vi "HapticSPM_force_only.vi"() -> ()   [LabVIEW 2023]
uses:
  HapticSPM_write Folder/Program Files/National Instruments/LabVIEW 2022/user.lib/Haptic Prog Interface/Haptic Prog Interface.lvlib
  Haptic-Programming-Interface/src/x64/Debug/Haptic Programming Interface.dll
panel:
  out "Potential vs Distance":cluster{dbl[], dbl[]}(graph)
  out "Force vs Distance":cluster{dbl[], dbl[]}(graph)
  in  "Suggested Settings":bool=TRUE
  out "Z-Position":dbl caption="Numeric" format="%#.17p"
  out "Force":dbl(knob) scale=-3.0..3.0
  in  "Function":string(combo)="2" caption="Combo Box"
  in  "k":dbl=1.0 caption="Numeric" step=0.1 format="%.1g"
  in  "Setpoint":dbl=1e-10 caption="Numeric" step=1e-11 format="%.0p"
  in  "Gain":dbl=1.0 caption="Numeric" format="%.1g"
  # "Super Ultra Mega Haptic SPM Controller 3000"
  # "Signal"
  # "Height"
  # "Force"
  # "Force"
  # "Move pen in all three dimensions to calibrate before feeling surface\n\nClick \"enter\" to turn off recommended settings\n\nChange \"Setpoint\" and \"k\" parameters to adjust the feel of the force"
  # "Surface Scale"
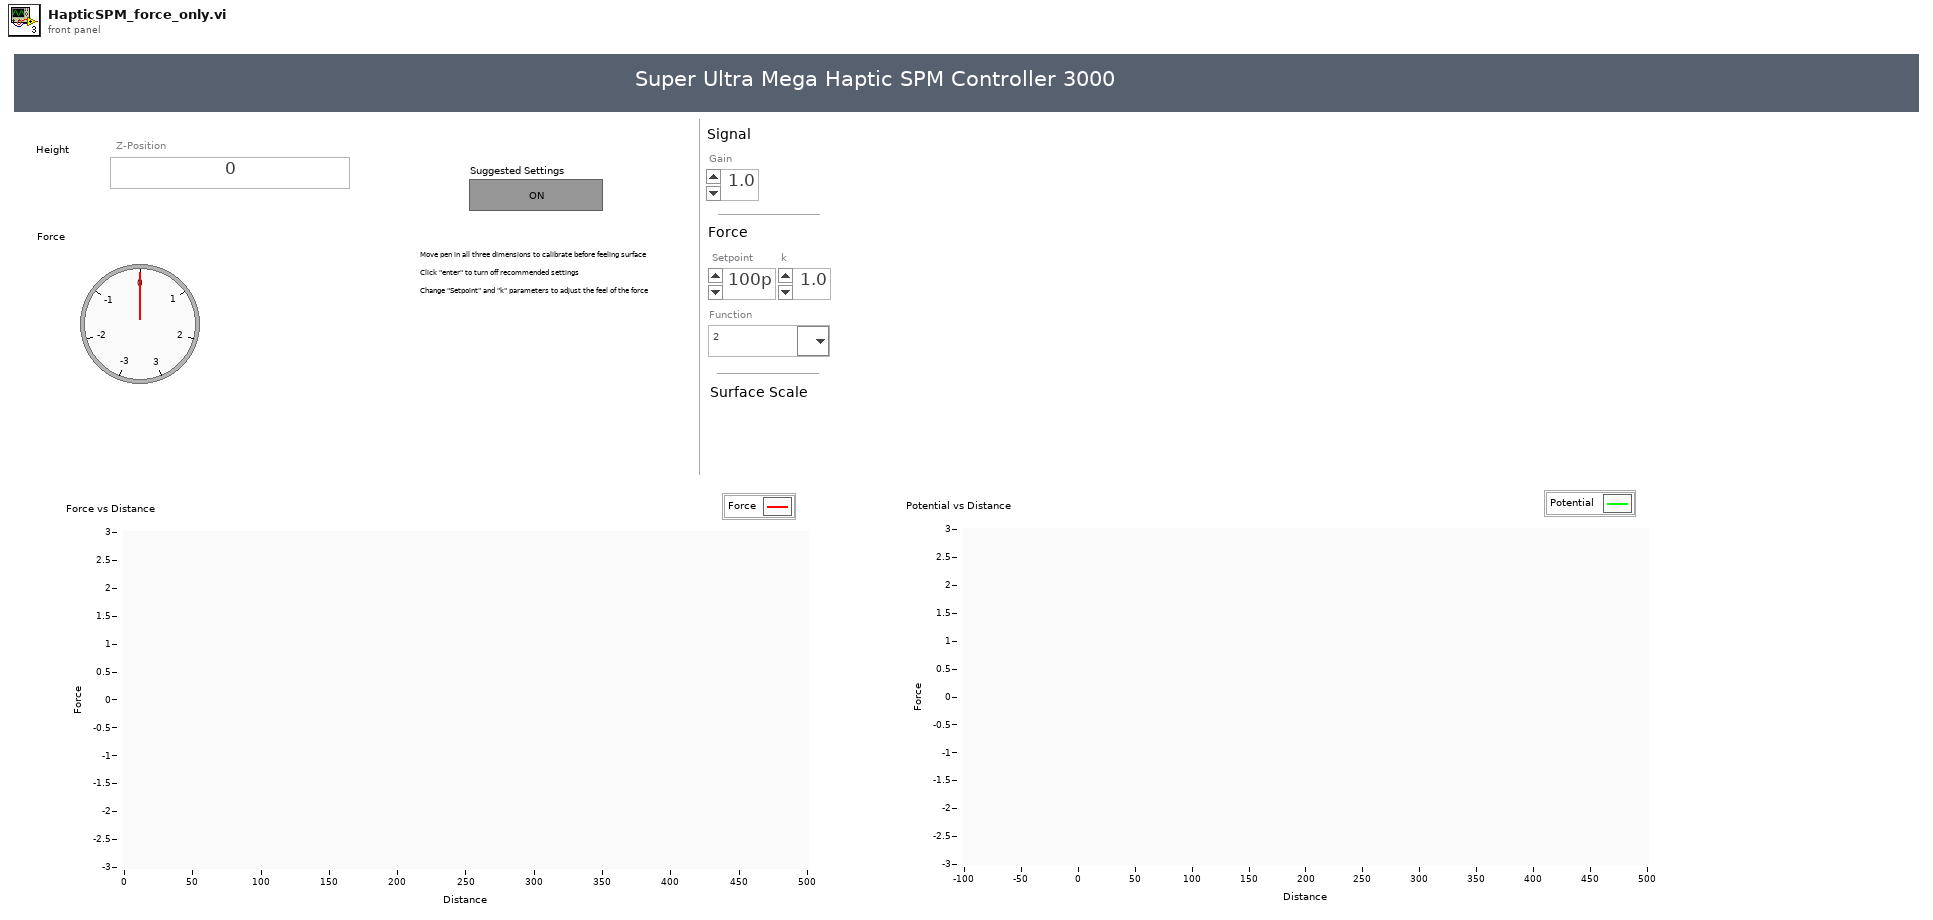
[diagram p1: front panel]
types:
  T1 = cluster{"Fx (N)":dbl, "Fy (N)":dbl, "Fz (N)":dbl}
  T2 = cluster{"kx (N/m)":dbl, "ky (N/m)":dbl, "kz (N/m)":dbl}
  T3 = cluster{"X Drag":bool, "Y Drag":bool, "Z Drag":bool}
  T4 = cluster{"x (mm)":dbl, "y (mm)":dbl, "z (mm)":dbl}
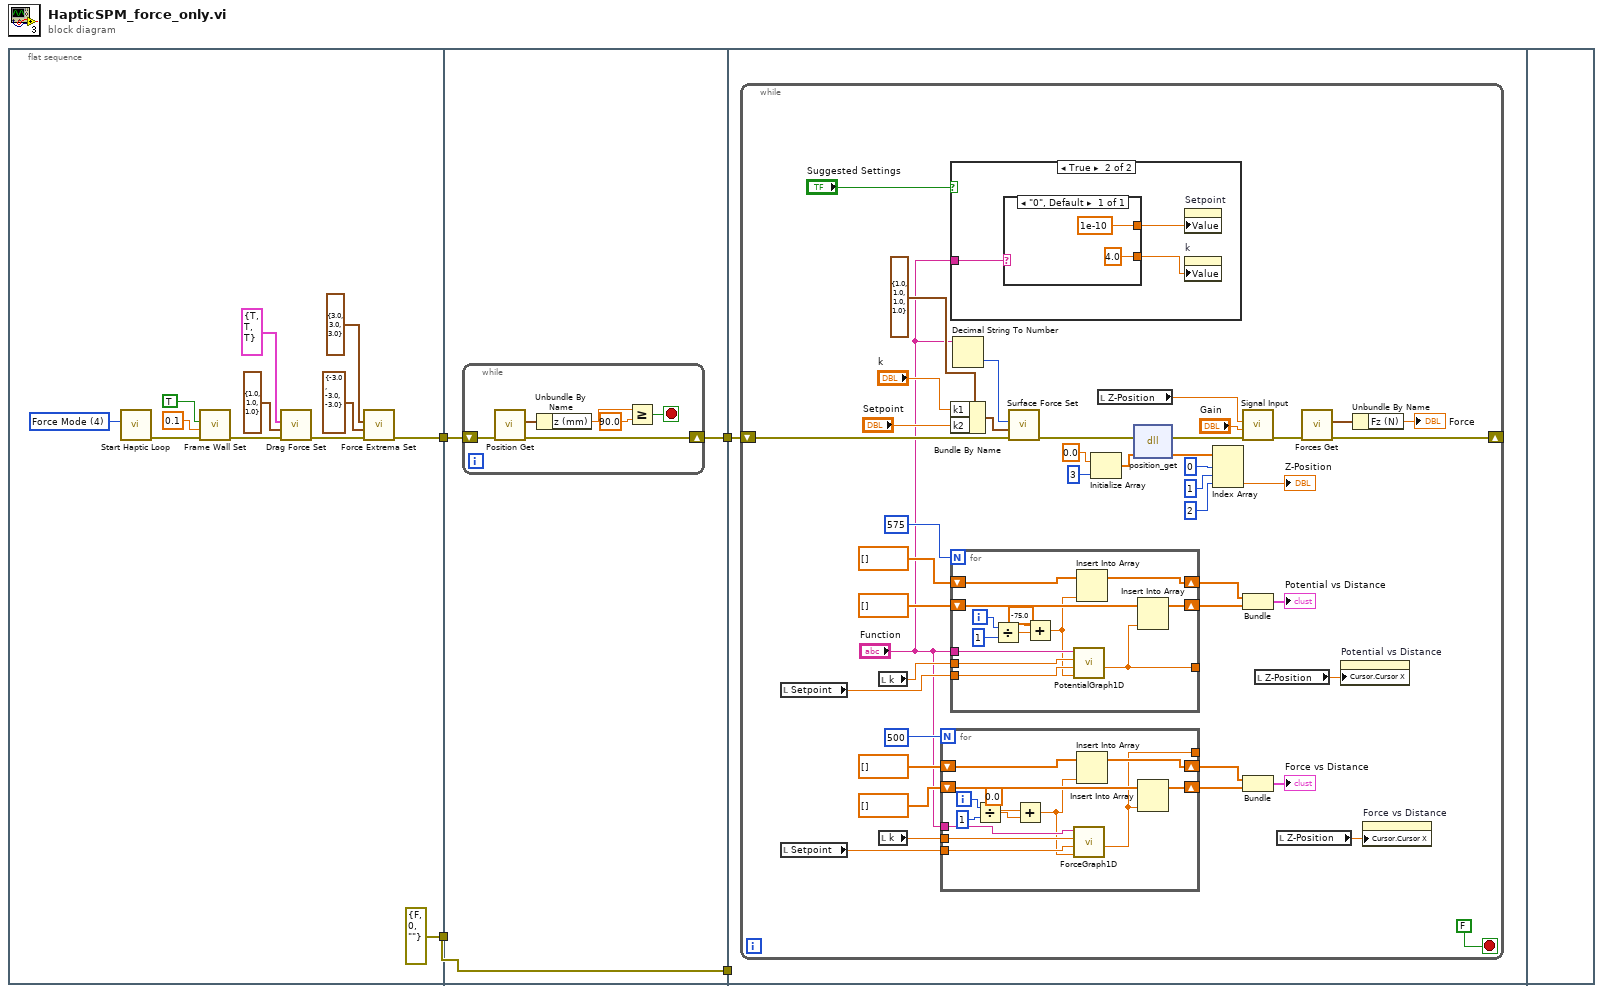
[diagram p0: block diagram]
diagram:
  n1 = flat-sequence {
    tunnel: [w14] -> w4
    tunnel: [errorcluster {"status"=FALSE, "code"=0, "source"=""} ("error out")] -> w1
    tunnel: w4 -> [w19]
    tunnel: [w18] -> w3
    tunnel: [w17] -> w2
    tunnel: w1 -> [w17]
    tunnel: w3 -> [w26]
    tunnel: w2 -> [_]
    frame #0 {
      w16 = u16 4 items=["Custom Mode", "Read Mode", "Write Mode", "Virtual Mode", "Force Mode"] ("Mode Selection")
      n2 = call "Start Haptic Loop.vi"("Mode Selection"=w16) -> ("error out"=w7:errorcluster)  [unwired: 10 in]
      n3 = call "Frame Wall Set.vi"("error in (no error)"=w7, "Wall Stiffness (N/m)"=0.1 ("Wall Stiffness"), "Restrict to Frame"=TRUE) -> ("error out"=w6:errorcluster)  [unwired: 8 in]
      n4 = call "Drag Force Set.vi"("error in (no error)"=w6, "Drag Coefficients (N/m)"=T2 {"kx (N/m)"=1.0, "ky (N/m)"=1.0, "kz (N/m)"=1.0} ("Drag Coefficients"), "Drag Force Toggles"=T3 {"X Drag"=TRUE, "Y Drag"=TRUE, "Z Drag"=TRUE}) -> ("error out"=w15:errorcluster)  [unwired: 8 in]
      n5 = call "Force Extrema Set.vi"("error in (no error)"=w15, "Minimum Force (N)"=T1 {"Fx (N)"=-3.0, "Fy (N)"=-3.0, "Fz (N)"=-3.0} ("Minimum Force"), "Maximum Force (N)"=T1 {"Fx (N)"=3.0, "Fy (N)"=3.0, "Fz (N)"=3.0} ("Maximum Force")) -> ("error out"=w14:errorcluster)  [unwired: 8 in]
    }
    frame #1 {
      n6 = while {
        shift-right: [w24] -> w18
        shift-left: w19 -> [w25]
        stop <- w20 stop-if-true
        n7 = call "Position Get.vi"("error in (no error)"=w25) -> ("error out"=w24:errorcluster, "Position"=w23:T4)  [unwired: 9 in]
        n8 = Unbundle By Name(w23) -> ("z (mm)"=w22:dbl)
        n9 = Greater Or Equal?(x=w22, y=90.0) -> (x >= y?=w20:bool)
      }
    }
    frame #2 {
      n10 = while {
        shift-right: [w39] -> _
        shift-left: w26 -> [w69]
        stop <- FALSE stop-if-true
        n11 = local read "Setpoint"() -> (w29:dbl)
        n12 = local read "Setpoint"() -> (w50:dbl)
        n13 = local read "k"() -> (w30:dbl)
        n14 = local read "k"() -> (w51:dbl)
        n15 = for {
          N: 500 -> [_]
          shift-right: [w95] -> w56
          shift-left: dbl[] [] -> [w93]
          shift-right: [w94] -> w57
          shift-left: dbl[] [] -> [w92]
          tunnel: "Function" -> [w88]
          tunnel: [w91] -> _
          tunnel: w50 -> [w90]
          tunnel: w51 -> [w89]
          i -> [w86]
          n16 = Divide(x=w86, y=1) -> (x/y=w85:dbl)
          n17 = Add(x=0.0, y=w85) -> (x+y=w83:dbl)
          n18 = call "ForceGraph1D.vi"("number"=w83, "Setpoint"=w90, "k"=w89, "Function"=w88) -> ("force"=w91:dbl)  [unwired: 7 in]
          n19 = Insert Into Array(array=w92, new element=w83) -> (w94:dbl[])  [unwired: 1 in]
          n20 = Insert Into Array(array=w93, new element=w91) -> (w95:dbl[])  [unwired: 1 in]
        }
        n21 = case shown="True" "Suggested Settings" {
          tunnel: "Function" -> [_ w98]
          frame False {
          }
          frame True {
            n22 = case shown="\"0\", Default" w98 {
              tunnel: [4.0] -> w97
              tunnel: [1e-10] -> w96
              frame "0", Default {
              }
            }
            n23 = property on="Setpoint" class="DigNum (strict)"("Value"=w96) -> ()  [unwired: 2 in, 2 out]
            n24 = property on="k" class="DigNum (strict)"("Value"=w97) -> ()  [unwired: 2 in, 2 out]
          }
        }
        n25 = Bundle By Name(cluster=cluster{"k1":dbl, "k2":dbl, "k3":dbl, "k4":dbl} {"k1"=1.0, "k2"=1.0, "k3"=1.0, "k4"=1.0} ("Force Constants"), "k1"="k", "k2"="Setpoint") -> (w65:cluster{"k1":dbl, "k2":dbl, "k3":dbl, "k4":dbl})
        n26 = for {
          N: 575 -> [_]
          shift-right: [w82] -> w35
          shift-left: dbl[] [] -> [w80]
          shift-right: [w81] -> w36
          shift-left: dbl[] [] -> [w79]
          tunnel: "Function" -> [w75]
          tunnel: [w78] -> _
          tunnel: w29 -> [w77]
          tunnel: w30 -> [w76]
          i -> [w73]
          n27 = Divide(x=w73, y=1) -> (x/y=w72:dbl)
          n28 = Add(x=-75.0, y=w72) -> (x+y=w70:dbl)
          n29 = call "PotentialGraph1D.vi"("number"=w70, "Setpoint"=w77, "k"=w76, "Function"=w75) -> ("potential"=w78:dbl)  [unwired: 7 in]
          n30 = Insert Into Array(array=w79, new element=w70) -> (w81:dbl[])  [unwired: 1 in]
          n31 = Insert Into Array(array=w80, new element=w78) -> (w82:dbl[])  [unwired: 1 in]
        }
        n32 = Decimal String To Number(string="Function") -> (number=w62:i32)  [unwired: 2 in, 1 out]
        n33 = call "Surface Force Set.vi"("error in (no error)"=w69, "Force Constants"=w65, "Force Settings"=w62) -> ("error out"=w45:errorcluster)  [unwired: 8 in]
        n34 = Initialize Array(0.0 ("element"), 3 ("dimension size")) -> (w46:dbl[])
        n35 = local read "Z-Position"() -> (w61:dbl)
        n36 = dll-call lib="C:/Users/cjwel/Documents/GitHub/Haptic-Programming-Interface/src/x64/Debug/Haptic Programming Interface.dll" fn="position_get"(error in=w45, "output"=w46) -> (error out=w44:errorcluster, "output"=w40:dbl[])  [unwired: 3 in, 1 out]
        n37 = Index Array(array=w40, index #1=0 ("index"), index #2=1 ("index"), index #3=2 ("index")) -> (element #3=→"Z-Position":dbl)  [unwired: 2 out]
        n38 = call "Signal Input.vi"("error in (no error)"=w44, "Gain"="Gain", "Signal"=w61) -> ("error out"=w68:errorcluster)  [unwired: 8 in]
        n39 = Bundle(w36, w35) -> (→"Potential vs Distance":cluster{dbl[], dbl[]})  [unwired: 1 in]
        n40 = Bundle(w57, w56) -> (→"Force vs Distance":cluster{dbl[], dbl[]})  [unwired: 1 in]
        n41 = local read "Z-Position"() -> (w27:dbl)
        n42 = local read "Z-Position"() -> (w49:dbl)
        n43 = call "Forces Get.vi"("error in (no error)"=w68) -> ("error out"=w39:errorcluster, "Force (N)"=w60:T1)  [unwired: 9 in]
        n44 = property on="Potential vs Distance" class="XYGraph (strict)"("Cursor.Cursor X"=w27) -> ()  [unwired: 2 in, 2 out]
        n45 = Unbundle By Name(w60) -> ("Fz (N)"=→"Force":dbl)
        n46 = property on="Force vs Distance" class="XYGraph (strict)"("Cursor.Cursor X"=w49) -> ()  [unwired: 2 in, 2 out]
      }
    }
    frame #3 {
    }
  }
